vi "Init.vi"(8 "error in (no error)":errorcluster, 9 "Config File Path":path=path "", 10 "Name":string, 11 "Mock Worker In":refnum<class "Mock Work Dispatcher.lvclass">) -> (0 "error out":errorcluster, 3 "Mock Worker Out":refnum<class "Mock Work Dispatcher.lvclass">)   [LabVIEW 2020, in "Mock Work Dispatcher.lvclass"]
doc: "Initialize the class and creates necessary references. Anything initialized here is released in the Clear.vi method."
uses:
  Mock Work Dispatcher.lvclass
  Mock Work Dispatcher.lvclass/Mock Work Dispatcher.ctl
  <vilib>/Asteme/Triarc Framework/Base/Base.lvclass
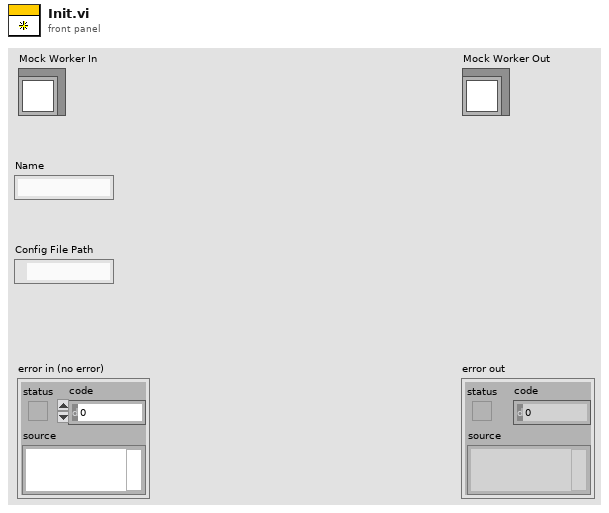
[diagram p1: front panel]
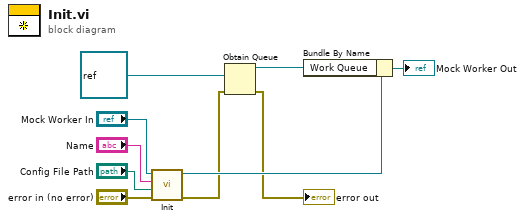
[diagram p0: block diagram]
diagram:
  n1 = call-parent "Init.vi"("error in (no error)"="error in (no error)", "Config File Path"="Config File Path", "Name"="Name", "Base In"="Mock Worker In") -> ("error out"=w2:errorcluster, "Base Out"=w10:refnum<class "Mock Work Dispatcher.lvclass">)  [unwired: 6 in]
  n2 = Obtain Queue(element data type=refnum<class> refnum ("LabVIEW Object"), error in (no error)=w2) -> (queue out=w3:refnum<queue>, error out=→"error out":errorcluster)  [unwired: 3 in, 1 out]
  n3 = Bundle By Name(cluster=w10, "Work Queue"=w3) -> (→"Mock Worker Out":refnum<class "Mock Work Dispatcher.lvclass">)
